vi "try_Zoom.vi"() -> ()   [LabVIEW 2020]
uses:
  <vilib>/Analysis/NI_AALBase.lvlib
panel:
  out "XY Graph":cluster{dbl[], dbl[]}[](graph)
  in  "Trigger":bool
  out "Write Buffer Status":dbl(graph)
  # "Zoom Demo"
  # "See the block diagram."
  # "Close this VI when you are done with the demo."
  # "You do not need to save changes to this VI."
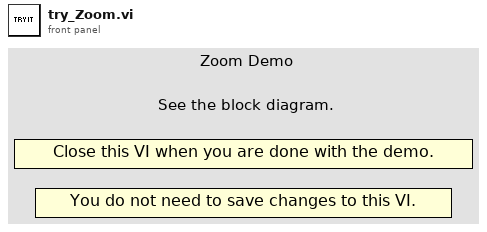
[diagram p1: front panel]
types:
  T1 = enum16{"open", "open or create", "create or replace", "create", "open (read-only)"}
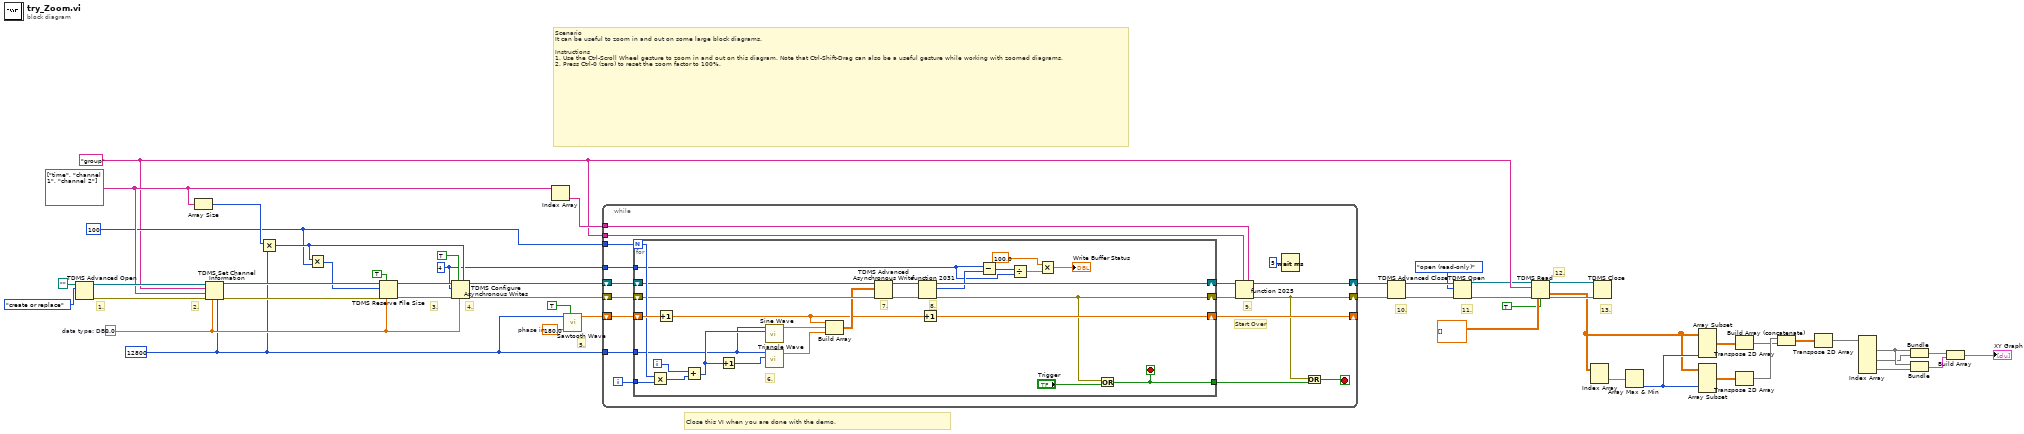
[diagram p0: block diagram]
diagram:
  w32 = 100 ("Pre-Trigger [number of samples]")
  w29 = 12800 ("Number of Samples")
  w38 = 180.0  # phase in
  w9 = u32 4 ("number of buffers (4)")
  w44 = 0.0  # data type: DBL
  w35 = string[] ["time", "channel 1", "channel 2"] ("channel name(s)")
  w25 = "group" ("group name (Untitled)")
  # "13."
  # "12."
  # "11."
  # "10."
  # "5."
  # "4."
  # "1."
  # "3."
  # "2."
  # "Close this VI when you are done with the demo."
  # "Scenario\nIt can be useful to zoom in and out on some large block diagrams.\n\nInstructions\n1. Use the Ctrl-Scroll Wheel gesture to zoom in and out on this diagram. Note that Ctrl-Shift-Drag can also be a useful gesture while working with zoomed diagrams.\n2. Press Ctrl-0 (zero) to reset the zoom factor to 100%."
  n1 = TDMS Advanced Open(10:T1."create or replace" ("operation (0:open)"), 11:path "") -> (0:w50:errorcluster, 3:w49:refnum<k34>)  [unwired: 3 in, 1 out]
  n2 = Array Size(array=w35) -> (size(s)=w34:i32)
  n3 = TDMS Set Channel Information(4:w29, 6:w44, 8:w50, 9:w35, 10:w25, 11:w49) -> (0:w48:errorcluster, 3:w47:refnum<k34>)  [unwired: 1 in]
  n4 = Multiply(x=w34, y=w29) -> (x*y=w33:i32)
  n5 = Multiply(x=w33, y=w32) -> (x*y=w31:i32)
  n6 = TDMS Reserve File Size(6:w44, 7:TRUE ("append? (T)"), 8:w48, 10:w31, 11:w47) -> (0:w46:errorcluster, 3:w45:refnum<k34>)
  n7 = TDMS Configure Asynchronous Writes(5:w33, 6:w44, 7:TRUE ("pre-allocate? (F)"), 8:w46, 10:w9, 11:w45) -> (0:w7:errorcluster, 3:w39:refnum<k34>)  [unwired: 1 in]
  n8 = Index Array(array=w35) -> (element=w40:string)  [unwired: 1 in]
  n9 = call <vilib>:"Sawtooth Wave.vi"("samples"=w29, "phase in"=w38, "reset phase"=TRUE) -> ("sawtooth wave"=w37:dbl[])  [unwired: 2 in, 2 out]
  n10 = while {
    tunnel: w25 -> [w68]
    tunnel: w40 -> [w67]
    shift-right: [w58] -> w41
    shift-left: w39 -> [w66]
    shift-right: [w52] -> w42
    shift-left: w7 -> [w65]
    shift-right: [w61] -> _
    shift-left: w37 -> [w62]
    tunnel: w29 -> [w59]
    tunnel: w32 -> [w57]
    tunnel: w9 -> [w54]
    i -> [w60]
    stop <- w56 stop-if-true
    # "9."
    # "Start Over"
    n11 = for {
      N: w57 -> [w94]
      shift-right: [w76] -> w63
      shift-left: w66 -> [w89]
      shift-right: [w69] -> w64
      shift-left: w65 -> [w88]
      shift-right: [w80] -> w61
      shift-left: w62 -> [w95]
      tunnel: w60 -> [w93]
      tunnel: w59 -> [w83]
      tunnel: [w84] -> w55
      tunnel: w54 -> [w73]
      i -> [w91]
      stop <- w84 stop-if-true
      # "8."
      # "7."
      # "6."
      n12 = Multiply(x=w94, y=w93) -> (x*y=w92:i32)
      n13 = Increment(x=w95) -> (x+1=w79:dbl[])
      n14 = Add(x=w91, y=w92) -> (x+y=w90:i32)
      n15 = Increment(x=w90) -> (x+1=w82:i32)
      n16 = call <vilib>:"Sine Wave.vi"("samples"=w83, "amplitude"=w90) -> ("sine wave"=w87:dbl[])  [unwired: 3 in, 2 out]
      n17 = call <vilib>:"Triangle Wave.vi"("samples"=w83, "amplitude"=w82) -> ("triangle wave"=w81:dbl[])  [unwired: 3 in, 2 out]
      n18 = Build Array(w79, w87, w81) -> (w86:dbl[][])
      n19 = TDMS Advanced Asynchronous Write(8:w88, 10:w86, 11:w89) -> (0:w78:errorcluster, 3:w77:refnum<k34>)
      n20 = fn#2031(8:w78, 11:w77) -> (0:w69:errorcluster, 2:w75:u32, 3:w76:refnum<k34>)
      n21 = Increment(x=w79) -> (x+1=w80:dbl[])
      n22 = Subtract(x=w73, y=w75) -> (x-y=w74:u32)
      n23 = Divide(x=w74, y=w73) -> (x/y=w72:dbl)
      n24 = Multiply(x=100.0, y=w72) -> (x*y=→"Write Buffer Status":dbl)
      n25 = Or(x=w69, y="Trigger") -> (x .or. y?=w84:bool)
    }
    n26 = fn#2025(5:w67, 7:w68, 8:w64, 11:w63) -> (0:w52:errorcluster, 3:w58:refnum<k34>)  [unwired: 2 in]
    n27 = Wait (ms)(milliseconds to wait=u32 5) -> ()  [unwired: 1 out]
    n28 = Or(x=w52, y=w55) -> (x .or. y?=w56:bool)
  }
  n29 = TDMS Advanced Close(8:w42, 11:w41) -> (0:w26:errorcluster, 3:w28:path)  [unwired: 2 in]
  n30 = TDMS Open(8:w26, 10:T1."open (read-only)" ("operation (0:open)"), 11:w28) -> (0:w6:errorcluster, 3:w5:refnum<k34>)  [unwired: 4 in]
  n31 = TDMS Read(0:w5, 5:w25, 11:w6, 12:dbl[][] [] ("sawtooth wave"), 13:TRUE ("return channels in file order? (F)")) -> (4:w21:refnum<k34>, 10:w2:dbl[][], 15:w20:errorcluster)  [unwired: 3 in, 3 out]
  n32 = Index Array(array=w2) -> (element=w23:dbl[])  [unwired: 2 in]
  n33 = TDMS Close(8:w20, 11:w21) -> ()  [unwired: 2 out]
  n34 = Array Max & Min(array=w23) -> (min index (indices)=w22:i32)  [unwired: 3 out]
  n35 = Array Subset(array=w2, length (col)=w22) -> (w15:dbl[][])  [unwired: 3 in]
  n36 = Array Subset(array=w2, index (col)=w22) -> (w14:dbl[][])  [unwired: 3 in]
  n37 = Transpose 2D Array(2D array=w15) -> (transposed array=w11:dbl[][])
  n38 = Transpose 2D Array(2D array=w14) -> (transposed array=w12:dbl[][])
  n39 = Build Array (concatenate)(w12, w11) -> (w13:dbl[][])
  n40 = Transpose 2D Array(2D array=w13) -> (transposed array=w10:dbl[][])
  n41 = Index Array(array=w10) -> (element #1=w19:dbl[], element #2=w4:dbl[], element #3=w3:dbl[])  [unwired: 6 in]
  n42 = Bundle(w19, w4) -> (w17:cluster{dbl[], dbl[]})  [unwired: 1 in]
  n43 = Bundle(w19, w3) -> (w18:cluster{dbl[], dbl[]})  [unwired: 1 in]
  n44 = Build Array(w17, w18) -> (→"XY Graph":cluster{dbl[], dbl[]}[])
